vi "ElectrodesLabelsToPickeringChannels.vi"(8 "error in (no error)":errorcluster, 9 "Labels":u16[](array[ring]) items=["", "I+", "I-", "V1", "V2", "V3", "Vsg"], 10 "Electrodes":T1(array[ring])) -> (0 "error out":errorcluster, 1 "Y Channel Array":string[][](array[string]), 2 "X Channel Array":string[](array[string]))   [LabVIEW 2016, in "Transport.lvclass"]
uses:
  Transport.lvclass
  levylab_inst_pickering/lvsrc/SMOs/pickering/pickering.lvclass
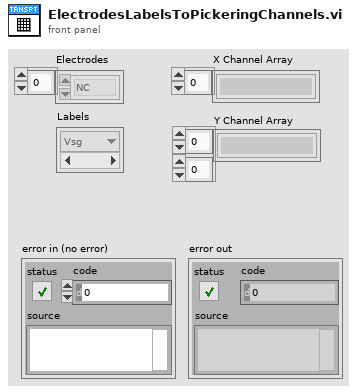
[diagram p1: front panel]
types:
  T1 = enum16{"NC", "26", "27", "28", "1", "2", "3", "4", "5", "6", "7", "8", "9", "10", "11", "12", "13", "14", "15", "16", "17", "18", "19", "20", "21", "22", "23", "24", "25"}[]
  T2 = typedef "pickering.lvclass/PickeringConfig-Cluster.ctl" = cluster{"x config":T3, "y config":T4}
  T3 = typedef "pickering.lvclass/PickeringXConfig-Cluster.ctl" = cluster{"Electrode":enum16{"NC", "26", "27", "28", "1", "2", "3", "4", "5", "6", "7", "8", "9", "10", "11", "12", "13", "14", "15", "16", "17", "18", "19", "20", "21", "22", "23", "24", "25"}[], "X Channels":string[]}
  T4 = typedef "pickering.lvclass/PickeringYConfig-Cluster.ctl" = cluster{"Label":u16[], "Y Channels":string[][]}
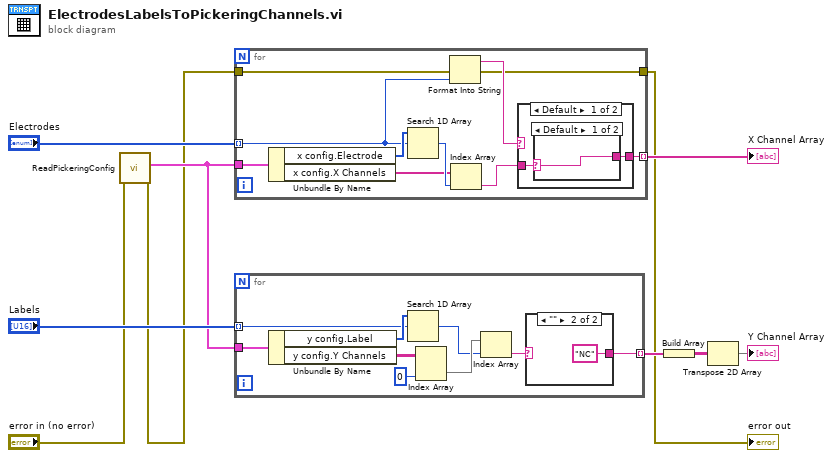
[diagram p0: block diagram]
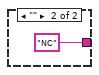
[diagram p3: hidden frame]
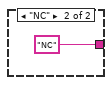
[diagram p4: hidden frame]
diagram:
  n1 = call "ReadPickeringConfig.vi"("error in (no error)"="error in (no error)") -> ("error out"=w4:errorcluster, "Pickering Config"=w5:T2)  [unwired: 9 in]
  n2 = for {
    tunnel: [w16] -> w9 mode=indexing
    tunnel: w5 -> [w19]
    tunnel: "Electrodes" -> [w15] mode=indexing
    tunnel: w4 -> [w12]
    tunnel: [w11] -> w3
    n3 = Unbundle By Name(w19) -> ("x config.Electrode"=w18:T1, "x config.X Channels"=w17:string[])
    n4 = Search 1D Array(1D array=w18, element=w15) -> (index of element=w20:i32)  [unwired: 1 in]
    n5 = Format Into String(error in=w12, w15) -> (resulting string=w13:string, error out=w11:errorcluster)  [unwired: 2 in]
    n6 = Index Array(array=w17, index=w20) -> (element=w14:string)
    n7 = case shown="Default" w13 {
      tunnel: [w21 "NC"] -> w16
      tunnel: w14 -> [w22 _]
      frame Default {
        n8 = case shown="Default" w22 {
          selector: w22 -> [w23 _]
          tunnel: [w23 "NC"] -> w21
          frame Default {
          }
          frame "" {
          }
        }
      }
      frame "NC" {
      }
    }
  }
  "error out" <- w3
  "X Channel Array" <- w9
  n9 = for {
    tunnel: w5 -> [w34]
    tunnel: "Labels" -> [w32] mode=indexing
    tunnel: [w26] -> w7 mode=indexing
    n10 = Unbundle By Name(w34) -> ("y config.Label"=w33:u16[], "y config.Y Channels"=w30:string[][])
    n11 = Search 1D Array(1D array=w33, element=w32) -> (index of element=w27:i32)  [unwired: 1 in]
    n12 = Index Array(array=w30, index (col)=0 ("disabled index (col)")) -> (element=w28:string[])  [unwired: 1 in]
    n13 = Index Array(array=w28, index=w27) -> (element=w29:string)
    n14 = case shown="\"\"" w29 {
      selector: w29 -> [w35 _]
      tunnel: [w35 "NC"] -> w26
      frame Default {
      }
      frame "" {
      }
    }
  }
  n15 = Build Array(w7) -> (w6:string[][])
  n16 = Transpose 2D Array(2D array=w6) -> (transposed array=→"Y Channel Array":string[][])
